vi "Create checking list.vi"() -> (3 "Stations":string[](array[string]))   [LabVIEW 2025, in "MES Interlcok.lvlib"]
uses:
  MES Interlcok.lvlib
  <vilib>/Utility/file.llb/Read Delimited Spreadsheet (string).vi
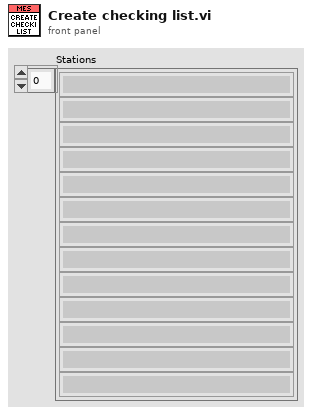
[diagram p1: front panel]
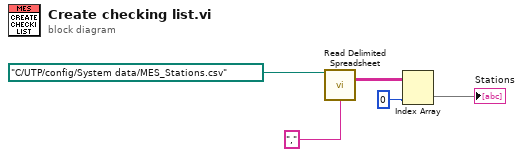
[diagram p0: block diagram]
diagram:
  n1 = call-poly <vilib>:"Read Delimited Spreadsheet.vi"("file path (dialog if empty)"=path "C:/UTP/config/System data/MES_Stations.csv", "delimiter (\\t)"="," ("delimiter (\\t)")) -> ("all rows"=w3:string[][])  [unwired: 8 in, 5 out]
  n2 = Index Array(array=w3, index (col)=0) -> (element=→"Stations":string[])  [unwired: 1 in]
